vi "case_selector.vi"(0 "kalibruj":bool, 1 "Terminal_Config":bool, 2 "bcfg in":bool, 5 "SAVE":bool, 7 "start in":bool, 9 "SAVE 2":bool, 11 "error in (no error)":errorcluster, 12 "START":bool) -> (4 "Boolean 3":bool, 6 "Boolean 2":bool, 8 "start out":bool, 10 "bcfg out":bool, 14 "Boolean":bool)   [LabVIEW 2013]
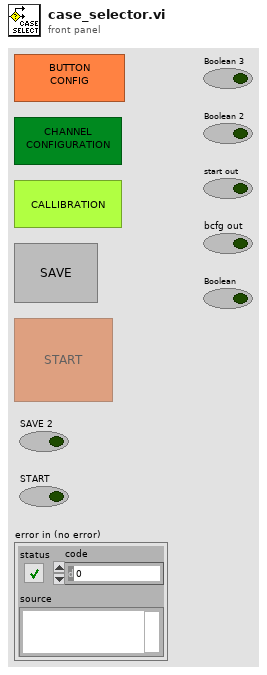
[diagram p1: front panel]
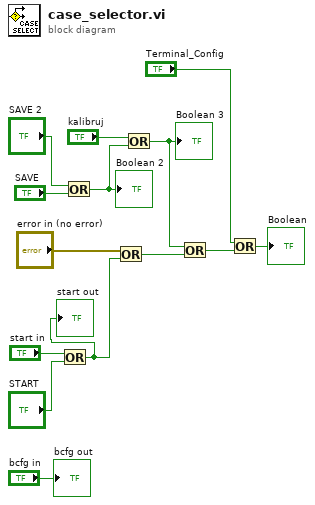
[diagram p0: block diagram]
diagram:
  n1 = Or(x="start in", y="START") -> (x .or. y?=w1:bool)
  "start out" <- w1
  n2 = Or(x="SAVE 2", y="SAVE") -> (x .or. y?=w7:bool)
  "Boolean 2" <- w7
  n3 = Or(x="error in (no error)", y=w1) -> (x .or. y?=w3:bool)
  n4 = Or(x="kalibruj", y=w7) -> (x .or. y?=w5:bool)
  "Boolean 3" <- w5
  n5 = Or(x=w5, y=w3) -> (x .or. y?=w11:bool)
  n6 = Or(x="Terminal_Config", y=w11) -> (x .or. y?=→"Boolean":bool)
  "bcfg out" <- "bcfg in"
